vi "Configure Analog Input Scale.vi"(0 "VISA resource name":refnum<visa-resource-name>, 1 "Analog Input (1)":i16=1, 2 "Scale Low (32.0)":dbl=32.0 format="%.2f", 3 "Scale High (1500.0)":dbl=1500.0 format="%.2f", 4 "Calibration Offset (0.0)":dbl format="%.2f", 5 "error in (no error)":errorcluster {"code" format="%.0x"}, 6 "Unit Address (1)":i16=1, 7 "Set Point Low Limit (32.0)":dbl=32.0 format="%.2f", 8 "Filter Time (0.0)":dbl format="%.2f", 9 "Set Point High Limit (1500.0)":dbl=1500.0 format="%.2f", 10 "Error Latch (0: Self Clear)":u16(ring) items=["Self Clear", "Latch"]) -> (14 "VISA resource name out":refnum<visa-resource-name>, 19 "error out":errorcluster {"code" format="%.0x"})   [LabVIEW 2010]
doc: "This VI is used to configure analog inputs."
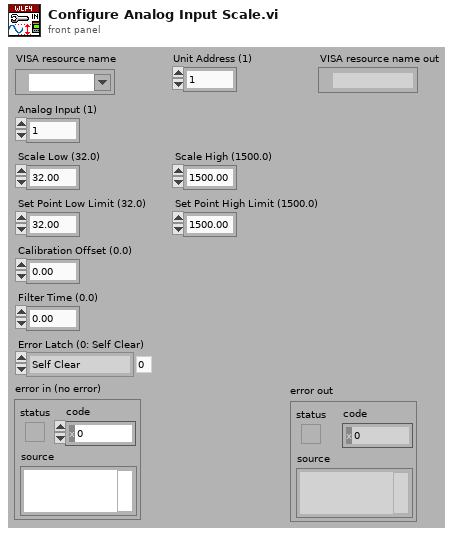
[diagram p1: front panel]
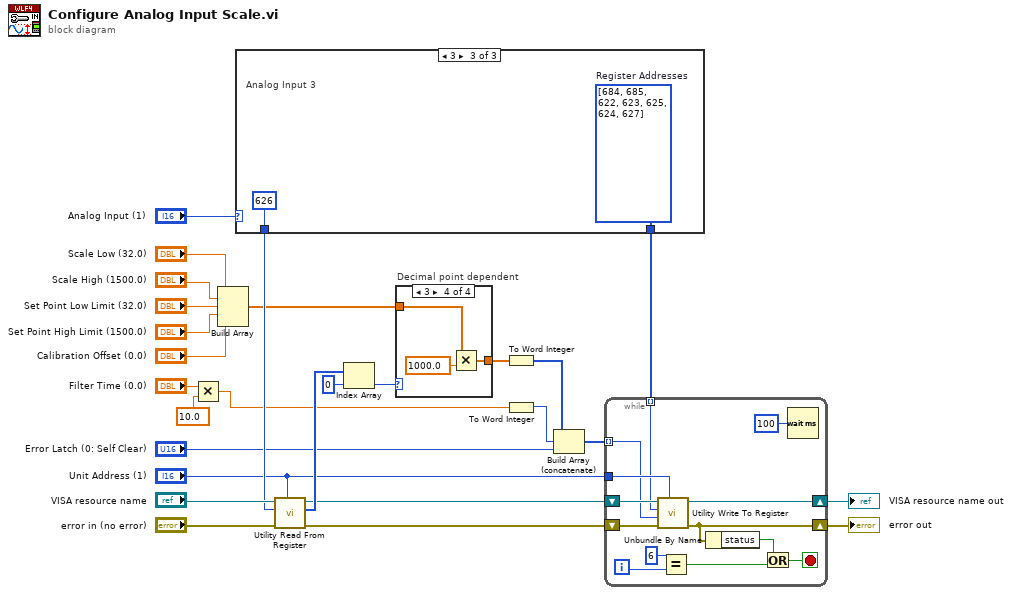
[diagram p0: block diagram]
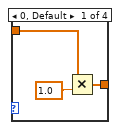
[diagram p2: hidden frame]
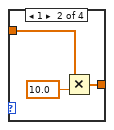
[diagram p3: hidden frame]
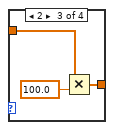
[diagram p4: hidden frame]
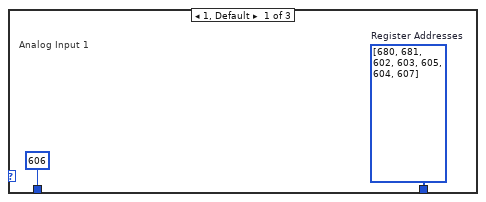
[diagram p5: hidden frame]
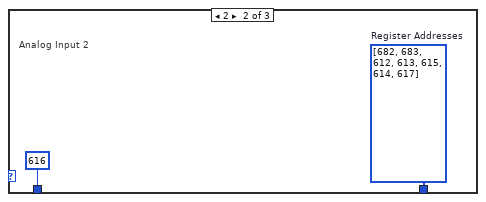
[diagram p6: hidden frame]
diagram:
  # "Decimal point dependent"
  n1 = Multiply(x="Filter Time (0.0)", y=10.0) -> (x*y=w5:dbl)
  n2 = Build Array("Scale Low (32.0)", "Scale High (1500.0)", "Set Point Low Limit (32.0)", "Set Point High Limit (1500.0)", "Calibration Offset (0.0)") -> (w10:dbl[])
  n3 = case shown="3" "Analog Input (1)" {
    tunnel: [w29 w31 w33] -> w20
    tunnel: [606 616 626] -> w15
    frame 1, Default {
      w29 = i32[] [680, 681, 602, 603, 605, 604, 607]  # Register Addresses
      # "Analog Input 1"
    }
    frame 2 {
      w31 = i32[] [682, 683, 612, 613, 615, 614, 617]  # Register Addresses
      # "Analog Input 2"
    }
    frame 3 {
      w33 = i32[] [684, 685, 622, 623, 625, 624, 627]  # Register Addresses
      # "Analog Input 3"
    }
  }
  n4 = call "Utility Read From Register.vi"("Unit Address (1)"="Unit Address (1)", "error in (no error)"="error in (no error)", "Register Address (0)"=w15, "VISA resource name"="VISA resource name") -> ("error out"=w18:errorcluster, "Data"=w23:i16[], "VISA resource name out"=w17:refnum<visa-resource-name>)  [unwired: 5 in]
  n5 = Index Array(array=w23, index=0) -> (element=w22:i16)
  n6 = case shown="3" w22 {
    tunnel: [w35 w38 w41 w44] -> w21
    tunnel: w10 -> [w34 w37 w40 w43]
    frame 0, Default {
      n7 = Multiply(x=w34, y=1.0) -> (x*y=w35:dbl[])
    }
    frame 1 {
      n8 = Multiply(x=w37, y=10.0) -> (x*y=w38:dbl[])
    }
    frame 2 {
      n9 = Multiply(x=w40, y=100.0) -> (x*y=w41:dbl[])
    }
    frame 3 {
      n10 = Multiply(x=w43, y=1000.0) -> (x*y=w44:dbl[])
    }
  }
  n11 = To Word Integer(number=w21) -> (16bit integer=w9:i16[])
  n12 = To Word Integer(number=w5) -> (16bit integer=w4:i16)
  n13 = Build Array (concatenate)(w9, w4, "Error Latch (0: Self Clear)") -> (w8:u16[])
  n14 = while {
    tunnel: "Unit Address (1)" -> [w58]
    shift-right: [w55] -> w27
    shift-left: w17 -> [w57]
    shift-right: [w50] -> w26
    shift-left: w18 -> [w56]
    tunnel: w20 -> [w53] mode=indexing
    tunnel: w8 -> [w52] mode=indexing
    i -> [w51]
    stop <- w47 stop-if-true
    n15 = call "Utility Write To Register.vi"("Unit Address (1)"=w58, "error in (no error)"=w56, "Data (0)"=w52, "Register Address (0)"=w53, "VISA resource name"=w57) -> ("error out"=w50:errorcluster, "VISA resource name out"=w55:refnum<visa-resource-name>)  [unwired: 5 in]
    n16 = Equal?(x=6, y=w51) -> (x = y?=w48:bool)
    n17 = Unbundle By Name(w50) -> ("status"=w49:bool)
    n18 = Or(x=w49, y=w48) -> (x .or. y?=w47:bool)
    n19 = Wait (ms)(milliseconds to wait=u32 100) -> ()  [unwired: 1 out]
  }
  "error out" <- w26
  "VISA resource name out" <- w27
